vi "Get Debug Flags.vi"(11 "Interface in":refnum<class "Engine Interface.lvclass">) -> (2 "FIFO Debug Flags":refnum<class "Debug Flags FIFO.lvclass">, 3 "Interface out":refnum<class "Engine Interface.lvclass">)   [LabVIEW 2017, in "Data Sharing Framework Engine.lvlib" / "Engine Interface.lvclass"]
uses:
  Engine Interface.lvclass
  Debug/Debug Flags FIFO/Debug Flags FIFO.lvclass
  Engine Interface.lvclass/Engine Interface.ctl
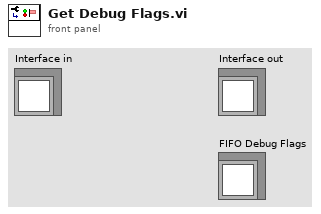
[diagram p1: front panel]
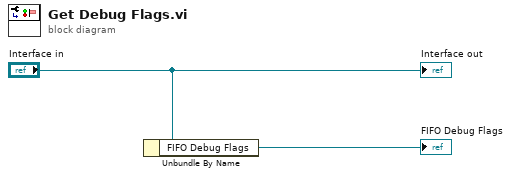
[diagram p0: block diagram]
diagram:
  n1 = Unbundle By Name("Interface in") -> ("FIFO Debug Flags"=→"FIFO Debug Flags":refnum<class "Debug Flags FIFO.lvclass">)
  "Interface out" <- "Interface in"
